vi "Config.File.Read.vi"(8 "error in":errorcluster, 11 "path":path) -> (0 "error out":errorcluster)   [LabVIEW 2016]
uses:
  Tma.lib/nlconfig.llb/fp2ini mode.ctl
  Config.Global.vi
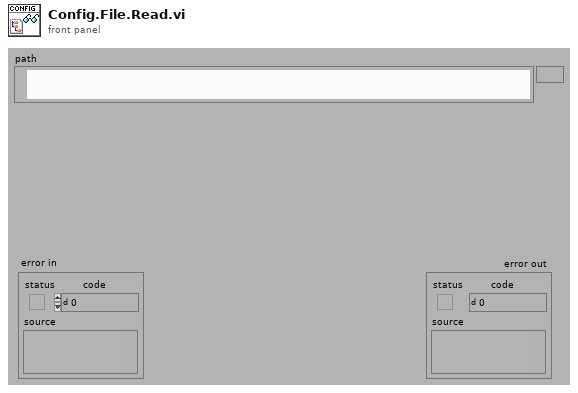
[diagram p1: front panel]
types:
  T1 = typedef "fp2ini mode.ctl" = enum16{"Read Controls", "Write Controls", "Write Indicators", "Read Indicators", "Write all", "Read all"}
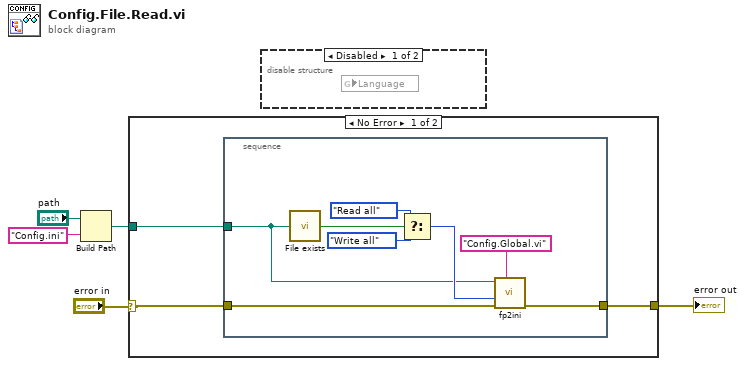
[diagram p0: block diagram]
diagram:
  n1 = Build Path(base path="path", name or relative path="Config.ini") -> (appended path=w1:path)
  n2 = case shown="No Error" "error in" {
    selector: "error in" -> [w8 w17]
    tunnel: [w7 w17] -> w5
    tunnel: w1 -> [w6 _]
    frame No Error {
      n3 = stacked-sequence {
        tunnel: w8 -> [w16]
        tunnel: [w15] -> w7
        tunnel: w6 -> [w9]
        frame #0 {
          n4 = call "File exists.vi"("file path"=w9) -> ("exists?"=w13:bool)  [unwired: 4 in]
          n5 = Select(t=fp2ini_mode."Read all" ("mode"), s=w13, f=fp2ini_mode."Write all" ("mode")) -> (s? t:f=w11:T1)
          n6 = call "fp2ini.vi"("vi-name (caller if empty)"="Config.Global.vi", "error in"=w16, "mode"=w11, "ini-file path"=w9) -> ("error out"=w15:errorcluster)  [unwired: 7 in]
        }
      }
    }
    frame Error {
    }
  }
  "error out" <- w5
  n7 = disable-structure shown="Disabled" {
    frame Disabled {
      n8 = global read "Config.Global.vi" "Language"() -> ()  [unwired: 1 in]
    }
    frame Enabled {
    }
  }
